vi "HFRR ADV v020 new software.vi"() -> ()   [LabVIEW 2025] (continued)
            n3927 = Concatenate Strings("\",\"ModelNumber\":\"" ("string"), w4967) -> (w4968:string)
            n3928 = Concatenate Strings("\",\"MachineRuntimeHours\":\"" ("string"), w4953) -> (w5071:string)
            n3929 = Concatenate Strings("\",\"MachineRuntimeCycles\":\"", w4962) -> (w5064:string)
            n3930 = Concatenate Strings(w5020, w5016) -> (w5050:string)
            n3931 = Concatenate Strings(w5019, w5006) -> (w5051:string)
            n3932 = Concatenate Strings(w5018, w4988) -> (w5049:string)
            n3933 = Concatenate Strings(w5070, w4968, w5071, w5064) -> (w5073:string)
            n3934 = Concatenate Strings(w5020, w5015) -> (w5047:string)
            n3935 = Concatenate Strings(w5019, w5005) -> (w5046:string)
            n3936 = Concatenate Strings(w5018, w4987) -> (w5048:string)
            n3937 = Concatenate Strings(w5020, w5014) -> (w5042:string)
            n3938 = Concatenate Strings(w5019, w5004) -> (w5043:string)
            n3939 = Concatenate Strings(w5018, w4986) -> (w5041:string)
            n3940 = Concatenate Strings(w5020, w5013) -> (w5039:string)
            n3941 = Concatenate Strings(w5019, w5003) -> (w5038:string)
            n3942 = Concatenate Strings(w5018, w4985) -> (w5040:string)
            n3943 = Concatenate Strings(w5050, w5051, w5049) -> (w5052:string)
            n3944 = Concatenate Strings(w5020, w5012) -> (w5029:string)
            n3945 = Concatenate Strings(w5019, w5002) -> (w5030:string)
            n3946 = Concatenate Strings(w5020, w5011) -> (w5026:string)
            n3947 = Concatenate Strings(w5019, w5001) -> (w5025:string)
            n3948 = Concatenate Strings(w5018, w4984) -> (w5028:string)
            n3949 = Concatenate Strings(w5018, w4983) -> (w5027:string)
            n3950 = Concatenate Strings("{\"SecretKey\":\"", w5067, w5073, "\",\"UUID\" : \"", w5062, "\",\"SensorInformation\":", "[{" ("string")) -> (w5000:string)
            n3951 = Concatenate Strings(w5047, w5046, w5048) -> (w5045:string)
            n3952 = Concatenate Strings(w5042, w5043, w5041) -> (w5044:string)
            n3953 = Concatenate Strings(w5039, w5038, w5040) -> (w5037:string)
            n3954 = Concatenate Strings(w5029, w5030, w5028) -> (w5031:string)
            n3955 = Concatenate Strings(w5026, w5025, w5027) -> (w5024:string)
            n3956 = Concatenate Strings(w5023, w5035, w5052, w4993) -> (w4999:string)
            n3957 = Concatenate Strings(w5023, w5034, w5045, w4993) -> (w4998:string)
            n3958 = Concatenate Strings(w5023, w5033, w5044, w4993) -> (w4997:string)
            n3959 = Concatenate Strings(w5023, w5032, w5037, w4993) -> (w4996:string)
            n3960 = Concatenate Strings(w5023, w5022, w5031, w4993) -> (w4995:string)
            n3961 = Concatenate Strings(w5023, w5021, w5024, "\"}" ("string")) -> (w4994:string)
            n3962 = Concatenate Strings(w5000, w4999, w4998, w4997, w4996, w4995, w4994, "]}" ("string")) -> (w4991:string)
            n3963 = local read "SEN.RUN HRS"() -> (w4958:dbl)
            n3964 = disable-structure shown="Disabled" {
              frame Disabled {
                n3965 = local read "state"() -> (w5077:string[])
                n3966 = Delete From Array(array=w5077, index=0) -> (array with subset deleted=w5075:string[])  [unwired: 1 in, 1 out]
                n3967 = for {
                  N: 6 -> [_]
                  tunnel: w5075 -> [w5088] mode=indexing
                  tunnel: [w5087] -> w5074 mode=indexing
                  n3968 = Equal?(x=w5088, y="Warning") -> (x = y?=w5084:bool)
                  n3969 = Equal?(x=w5088, y="Healthy") -> (x = y?=w5081:bool)
                  n3970 = Select(t="2" ("y"), s=w5084, f="3" ("y")) -> (s? t:f=w5079:string)
                  n3971 = Select(t="1" ("y"), s=w5081, f=w5079) -> (s? t:f=w5087:string)
                }
                "state1" <- w5074
              }
              frame Enabled {
              }
            }
            n3972 = stacked-sequence {
              tunnel: w4991 -> [w5099 _ _]
              tunnel: [_ _ w5115] -> _
              frame #0 {
                (unwired) FALSE ("convert eol (F)")
                w5101 = enum16{"start", "end", "current"}."start" ("pos mode (0:2)")
                n3973 = local read "Path"() -> (w5095:path)
                n3974 = Path To String(path=w5095) -> (string=w5107:string)
                n3975 = Concatenate Strings(w5107, "\\", "Sensor File Name") -> (w5108:string)
                n3976 = local write "standard output 2"(" ") -> ()
                n3977 = String To Path(string=w5108) -> (path=w5098:path)
                n3978 = call <vilib>:"Open_Create_Replace File.vi"("advisory dialog? (display:T)"=FALSE, "function (open:0)"=T32."create or replace", "file path"=w5098) -> ("error out"=w5111:errorcluster, "refnum"=w5110:refnum<file>)  [unwired: 5 in, 2 out]
                n3979 = Set File Position(refnum=w5110, from (0:start)=w5101, error in=w5111) -> (refnum out=w5091:refnum<file>, error out=w5090:errorcluster)  [unwired: 1 in]
                n3980 = Write to Binary File(file (use dialog)=w5091, data=" ", error in=w5090, 5:FALSE ("prepend array or string size? (T)")) -> (refnum out=w5102:refnum<file>, error out=w5103:errorcluster)  [unwired: 2 in, 1 out]
                n3981 = Set File Position(offset (in bytes) (0)=w5101, refnum=w5102, error in=w5103) -> (refnum out=w5094:refnum<file>, error out=w5093:errorcluster)  [unwired: 1 in]
                n3982 = Write to Binary File(file (use dialog)=w5094, data=w5099, error in=w5093, 5:FALSE ("prepend array or string size? (T)")) -> (error out=w5097:errorcluster)  [unwired: 2 in, 2 out]
                n3983 = flat-sequence {
                  tunnel: w5098 -> [w5113]
                  tunnel: w5097 -> [_]
                  frame #0 {
                    n3984 = call <vilib>:"Read Characters From File.vi"("file path (dialog if empty)"=w5113) -> ("character string"=→"Sensor Health JSON string":string)  [unwired: 5 in, 3 out]
                  }
                }
                "SinglePoint  2" <- w5099
              }
              frame #1 {
              }
              frame #2 {
                (unwired) "\"Stored\": true" ("string")
                n3985 = call <vilib>:"System Exec.vi"("run minimized? (F)"=TRUE, "wait until completion? (T)"=TRUE, "working directory"=path "C:/LAB-IQ-NXT", "command line"="C:\\LAB-IQ-NXT\\JPostH.bat") -> ("standard error"=→"Respose From Server 2":string, "standard output"=w5118:string)  [unwired: 4 in, 2 out]
                "standard output 2" <- w5118
                n3986 = Match Pattern(string=w5118, regular expression="JSONH Check String") -> (match substring=w5116:string, offset past match=w5115:i32)  [unwired: 1 in, 2 out]
                n3987 = Equal?(x=w5116, y="JSONH Check String") -> (x = y?=→"Upload \nConfirmed 2":bool)
              }
            }
            n3988 = Divide(x=w4958, y=3600.0 ("f")) -> (x/y=w4951:dbl)
            n3989 = local read "run time"() -> (w5008:string[])
            n3990 = Round To Nearest(number=w4951) -> (nearest integer value=w4950:dbl)
            n3991 = Number To Decimal String(number=w4950) -> (decimal integer string=w4949:string)  [unwired: 1 in]
            n3992 = Index Array(array="Sensor Information", index (col) #1=0 ("disabled index (col)"), index (col) #2=1 ("index (col)"), index (col) #3=2 ("index (col)"), index (col) #4=3 ("index (col)")) -> (element #1=→"Sensor name":string[], element #2=→"model num":string[], element #3=→"run time":string[], element #4=→"state":string[])  [unwired: 4 in]
            n3993 = Insert Into Array(array=w5008, index=1, new element #1=w4949, new element #2=w4949, new element #3=w4949, new element #4=w4949, new element #5=w4949, new element #6=w4949) -> (w4973:string[])
            "run" <- w4973
            n3994 = local read "out"() -> (w4955:string[])
            n3995 = local read "Sensor Information"() -> (w4975:string[][])
            n3996 = Replace Array Subset(array=w4975, new element #1=w4973, index (col) #1=2 ("disabled index (col)"), new element #2=w4955, index (col) #2=3 ("index (col)")) -> (w4974:string[][])  [unwired: 2 in]
            n3997 = local write "Sensor Information"(w4974) -> ()
          }
        }
        n3998 = case shown="True" w4922 {
          frame False {
          }
          frame True {
            n3999 = Equal?(x="FLAG", y=0.0) -> (x = y?=w4939:bool)
            n4000 = case shown="False" w4939 {
              frame False {
                n4001 = Get Date/Time In Seconds() -> (seconds since 1Jan1904=w4945:timestamp)
                n4002 = local read "START 2"() -> (w4943:dbl)
                n4003 = To Double Precision Float(number=w4945) -> (double precision float=w4944:dbl)
                n4004 = Subtract(x=w4944, y=w4943) -> (x-y=→"SENSOR TIME  2":dbl)
              }
              frame True {
                n4005 = Get Date/Time In Seconds() -> (seconds since 1Jan1904=w4947:timestamp)
                n4006 = To Double Precision Float(number=w4947) -> (double precision float=→"START 2":dbl)
                n4007 = local write "FLAG"(100.0 ("FLAG")) -> ()
              }
            }
          }
        }
        n4008 = disable-structure shown="Disabled" {
          disable-tunnel: w4925 -> [w4934 _]
          disable-tunnel: [w4933 _] -> w4924
          frame Disabled {
            n4009 = local read "Json St Flg"() -> (w4932:bool)
            n4010 = case shown="True" w4932 {
              tunnel: w4934 -> [w4935 w4937]
              tunnel: [w4935 w4936] -> w4933
              frame False {
              }
              frame True {
                n4011 = Increment(x=w4937) -> (x+1=w4936:dbl)
                "T cycle" <- w4936
                n4012 = local write "Json St Flg"(FALSE ("Json St Flg")) -> ()
              }
            }
          }
          frame Enabled {
          }
        }
        n4013 = local read "Quit"() -> (w4919:bool)
      }
    }
    frame Enabled {
    }
  }
  n4014 = stacked-sequence {
    tunnel: [w5317] -> w44
    frame #0 {
      w5317 = FALSE ("Upload \nConfirmed")
      n4015 = local write "Upload \nConfirmed"(w5317) -> ()
      n4016 = local write "St Str"("") -> ()
    }
  }
  n4017 = disable-structure shown="Disabled" {
    disable-tunnel: w44 -> [w5318 _]
    frame Disabled {
      n4018 = case shown="True" {
        selector: _ -> [_ _]
        tunnel: w5318 -> [_ w5319]
        frame False {
        }
        frame True {
          n4019 = while {
            tunnel: [w5325] -> _
            tunnel: w5319 -> [_]
            i -> [w5325]
            stop <- w5320 stop-if-true
            n4020 = local read "Json End Flg"() -> (w5324:bool)
            n4021 = Wait (ms)(milliseconds to wait=u32 20 ("Refresh Rate (ms)")) -> ()  [unwired: 1 out]
            n4022 = local read "refresh flag"() -> (w5321:bool)
            n4023 = local read "RUN"() -> (w5322:bool)
            n4024 = And(x=w5322, y=w5321) -> (x .and. y?=w5323:bool)
            n4025 = Or(x=w5323, y=w5324) -> (x .or. y?=w5326:bool)
            "AR Led" <- w5326
            n4026 = case shown="True" w5326 {
              frame False {
              }
              frame True {
                w5343 = "\",\""
                n4027 = local read "UUID"() -> (w5341:string)
                n4028 = local write "refresh flag"(FALSE ("refresh flag")) -> ()
                n4029 = local read "time"() -> (w5330:dbl)
                n4030 = Multiply(x=w5330, y=60.0) -> (x*y=w5329:dbl)
                n4031 = Concatenate Strings("UUID\" : \"", w5341, "\"}") -> (w5344:string)
                n4032 = Number To Fractional String(number=w5329, width (-)=i16 10, precision (6)=i16 4) -> (F-format string=w5358:string)  [unwired: 1 in]
                n4033 = Concatenate Strings("{", "\"Time\":\"", w5358, w5343) -> (w5353:string)
                n4034 = stacked-sequence {
                  tunnel: w5343 -> [w5406 w5414 w5421 w5429 w5437 w5446 w5453]
                  tunnel: [w5407 _ _ _ _ _ _] -> w5357
                  tunnel: [_ w5415 _ _ _ _ _] -> w5356
                  tunnel: [_ _ w5422 _ _ _ _] -> w5355
                  tunnel: [_ _ _ w5431 _ _ _] -> w5354
                  tunnel: w5344 -> [_ _ _ _ _ _ w5464]
                  tunnel: [_ _ _ _ _ _ w5463] -> w5340
                  tunnel: [_ _ _ _ _ w5443 _] -> w5339
                  tunnel: [_ _ _ _ w5436 _ _] -> w5338
                  frame #0 {
                    n4035 = local read "NORMAL LOAD"() -> (w5405:dbl)
                    n4036 = Number To Fractional String(number=w5405, width (-)=i16 10, precision (6)=i16 4) -> (F-format string=w5408:string)  [unwired: 1 in]
                    n4037 = Concatenate Strings("NormalLoad\":\"", w5408, w5406) -> (w5407:string)
                  }
                  frame #1 {
                    n4038 = local read "Temp"() -> (w5413:dbl)
                    n4039 = Number To Fractional String(number=w5413, width (-)=i16 10, precision (6)=i16 4) -> (F-format string=w5416:string)  [unwired: 1 in]
                    n4040 = Concatenate Strings("Temperature\":\"", w5416, w5414) -> (w5415:string)
                  }
                  frame #2 {
                    n4041 = local read "cof"() -> (w5419:dbl)
                    n4042 = Number To Fractional String(number=w5419, width (-)=i16 10, precision (6)=i16 4) -> (F-format string=w5423:string)  [unwired: 1 in]
                    n4043 = Concatenate Strings("FrictionalForce\":\"", w5423, w5421) -> (w5422:string)
                  }
                  frame #3 {
                    n4044 = local read "Set Hz"() -> (w5427:dbl)
                    n4045 = Multiply(x=w5427, y=60.0) -> (x*y=w5426:dbl)
                    n4046 = Number To Fractional String(number=w5426, width (-)=i16 10, precision (6)=i16 4) -> (F-format string=w5432:string)  [unwired: 1 in]
                    n4047 = Concatenate Strings("Speed\":\"", w5432, w5429) -> (w5431:string)
                  }
                  frame #4 {
                    n4048 = local read item#-1() -> (w5435)
                    n4049 = Number To Fractional String(number=w5435, width (-)=i16 10, precision (6)=i16 4) -> (F-format string=w5439:string)  [unwired: 1 in]
                    n4050 = Concatenate Strings("LinearDeformation\":\"", w5439, w5437) -> (w5436:string)
                  }
                  frame #5 {
                    n4051 = local read "AIR TEMP"() -> (w5442:dbl)
                    n4052 = local read "Json St Flg"() -> (w5444:bool)
                    n4053 = local read "Json End Flg"() -> (w5445:bool)
                    n4054 = Number To Fractional String(number=w5442, width (-)=i16 10, precision (6)=i16 4) -> (F-format string=w5448:string)  [unwired: 1 in]
                    n4055 = Concatenate Strings("Vibration\":\"", w5448, w5446) -> (w5443:string)
                    n4056 = And(x=w5444, y=w5445) -> ()  [unwired: 1 out]
                  }
                  frame #6 {
                    n4057 = local read "Json End Flg"() -> (w5452:bool)
                    n4058 = Get Date/Time In Seconds() -> (seconds since 1Jan1904=w5460:timestamp)
                    n4059 = local read "Json St Flg"() -> (w5451:bool)
                    n4060 = To Double Precision Float(number=w5460) -> (double precision float=w5459:dbl)
                    n4061 = Subtract(x=w5459, y=2082844800.0) -> (x-y=w5457:dbl)
                    n4062 = Number To Fractional String(number=w5457, width (-)=i16 12, precision (6)=i16 0) -> (F-format string=w5454:string)  [unwired: 1 in]
                    n4063 = case shown="True" w5452 {
                      tunnel: ["" w5467] -> w5461
                      tunnel: w5454 -> [_ w5468]
                      tunnel: w5453 -> [_ w5466]
                      frame False {
                      }
                      frame True {
                        n4064 = local write "Json End Flg"(FALSE ("Json St Flg")) -> ()
                        n4065 = Concatenate Strings("End\": \"", w5468, w5466) -> (w5467:string)
                      }
                    }
                    n4066 = case shown="True" w5451 {
                      tunnel: [w5471 w5474] -> w5462
                      tunnel: w5454 -> [_ w5475]
                      tunnel: w5453 -> [_ w5472]
                      frame False {
                        n4067 = local read "St Str"() -> (w5471:string)
                      }
                      frame True {
                        n4068 = Concatenate Strings("Start\":\"", w5475, w5472) -> (w5474:string)
                        "St Str" <- w5474
                        n4069 = local write "Json St Flg"(FALSE ("Json St Flg")) -> ()
                      }
                    }
                    n4070 = Concatenate Strings(w5462, w5461, w5464) -> (w5463:string)
                  }
                }
                n4071 = local read "FILE"() -> (w5332:string)
                n4072 = Concatenate Strings("\",\"OperatorID\":\"" ("string"), "Operator ID") -> (w5335:string)
                n4073 = Concatenate Strings("\",\"DatasetTitle\":\"" ("string"), w5332) -> (w5334:string)
                n4074 = Concatenate Strings("\",\"SerialNumber\":\"" ("string"), "Serial No") -> (w5364:string)
                n4075 = Concatenate Strings("\",\"ModelNumber\":\"" ("string"), "Model No") -> (w5363:string)
                n4076 = Concatenate Strings(w5364, w5363) -> (w5346:string)
                n4077 = Concatenate Strings("{\"SecretKey\":\"", "Secret Key", w5346, w5335, w5334, "\",\"Samples\":[") -> (w5351:string)
                n4078 = Concatenate Strings(w5353, w5357, w5356, w5355, w5354, w5338, w5339, w5340) -> (w5352:string)
                n4079 = Concatenate Strings(w5351, w5352, "]}") -> (w5350:string)
                n4080 = stacked-sequence {
                  tunnel: w5350 -> [w5379 _ _]
                  tunnel: [_ _ w5396] -> _
                  frame #0 {
                    (unwired) FALSE ("convert eol (F)")
                    w5381 = enum16{"start", "end", "current"}."start" ("pos mode (0:2)")
                    n4081 = Path To String(path="Path") -> (string=w5387:string)
                    n4082 = Concatenate Strings(w5387, "\\", "Data File Name") -> (w5389:string)
                    n4083 = local write "standard output"(" ") -> ()
                    n4084 = String To Path(string=w5389) -> (path=w5378:path)
                    n4085 = call <vilib>:"Open_Create_Replace File.vi"("advisory dialog? (display:T)"=FALSE, "function (open:0)"=T32."create or replace", "file path"=w5378) -> ("error out"=w5392:errorcluster, "refnum"=w5391:refnum<file>)  [unwired: 5 in, 2 out]
                    n4086 = Set File Position(refnum=w5391, from (0:start)=w5381, error in=w5392) -> (refnum out=w5372:refnum<file>, error out=w5371:errorcluster)  [unwired: 1 in]
                    n4087 = Write to Binary File(file (use dialog)=w5372, data=" ", error in=w5371, 5:FALSE ("prepend array or string size? (T)")) -> (refnum out=w5382:refnum<file>, error out=w5383:errorcluster)  [unwired: 2 in, 1 out]
                    n4088 = Set File Position(offset (in bytes) (0)=w5381, refnum=w5382, error in=w5383) -> (refnum out=w5375:refnum<file>, error out=w5374:errorcluster)  [unwired: 1 in]
                    n4089 = Write to Binary File(file (use dialog)=w5375, data=w5379, error in=w5374, 5:FALSE ("prepend array or string size? (T)")) -> (error out=w5377:errorcluster)  [unwired: 2 in, 2 out]
                    n4090 = flat-sequence {
                      tunnel: w5378 -> [w5394]
                      tunnel: w5377 -> [_]
                      frame #0 {
                        n4091 = call <vilib>:"Read Characters From File.vi"("file path (dialog if empty)"=w5394) -> ("character string"=→"JSON string":string)  [unwired: 5 in, 3 out]
                      }
                    }
                    "SinglePoint" <- w5379
                  }
                  frame #1 {
                  }
                  frame #2 {
                    (unwired) "\"Stored\": true" ("string")
                    n4092 = call <vilib>:"System Exec.vi"("run minimized? (F)"=TRUE, "wait until completion? (T)"=TRUE, "working directory"=path "C:/LAB-IQ-NXT", "command line"="C:\\LAB-IQ-NXT\\JPost.bat") -> ("standard error"=→"Respose From Server":string, "standard output"=w5399:string)  [unwired: 4 in, 2 out]
                    "standard output" <- w5399
                    n4093 = Match Pattern(string=w5399, regular expression="JSON Check String") -> (match substring=w5397:string, offset past match=w5396:i32)  [unwired: 1 in, 2 out]
                    n4094 = Equal?(x=w5397, y="JSON Check String") -> (x = y?=→"Upload \nConfirmed":bool)
                  }
                }
              }
            }
            n4095 = local read "Quit"() -> (w5320:bool)
          }
        }
      }
    }
    frame Enabled {
    }
  }
  n4096 = disable-structure shown="Disabled" {
    disable-tunnel: _ -> [w5482 _]
    frame Disabled {
      n4097 = while {
        shift-right: [w5490] -> w5478
        shift-left: _ -> [w5491]
        shift-right: [w5488] -> w5479
        shift-left: errorcluster {"status"=TRUE, "code"=0, "source"="Init"} ("error out") -> [w5489]
        shift-right: [w5486] -> _
        shift-left: "" -> [w5487]
        tunnel: [w5484] -> _
        tunnel: w5482 -> [_]
        i -> [w5484]
        stop <- w5483 stop-if-true
        n4098 = flat-sequence {
          tunnel: [w5492] -> w5485
          frame #0 {
            n4099 = Wait (ms)(milliseconds to wait=10.0 ("Delay")) -> (millisecond timer value=w5492:u32)
          }
        }
        n4100 = case shown="No Error" w5489 {
          selector: w5489 -> [w5522 w5641]
          tunnel: [w5505 w5643] -> w5490
          tunnel: [w5504 w5642] -> w5488
          tunnel: w5491 -> [w5523 w5635]
          tunnel: w5487 -> [w5503 w5634]
          tunnel: [w5502 w5634] -> w5486
          tunnel: w5485 -> [_ _]
          frame No Error {
            n4101 = Concatenate Strings("\r", "\n") -> (w5514:string)  [unwired: 1 in]
            n4102 = case shown="True" w5515 {
              tunnel: w5523 -> [w5547 w5554]
              tunnel: w5522 -> [w5546 w5553]
              tunnel: [w5547 w5552] -> w5521
              tunnel: [w5546 w5551] -> w5501
              tunnel: w5514 -> [_ w5550]
              frame False {
              }
              frame True {
                n4103 = VISA Write(VISA resource name=w5554, write buffer=w5550, error in (no error)=w5553) -> (VISA resource name out=w5552:refnum<visa-resource-name>, error out=w5551:errorcluster)  [unwired: 1 out]
                n4104 = local write "Read String"("") -> ()
                n4105 = local write item#-1(FALSE) -> ()
              }
            }
            n4106 = property class="Instr"(reference=w5521, error in=w5501) -> (reference out=w5520:refnum<visa-resource-name>, error out=w5519:errorcluster, "Serial Settings:Number of Bytes at Serial Port"=w5518:u32)
            n4107 = Greater?(x=w5518, y=u32 100) -> (0:w5516:bool)
            n4108 = case shown="True" w5516 {
              tunnel: w5520 -> [w5557 w5581]
              tunnel: w5519 -> [w5556 w5580]
              tunnel: w5518 -> [_ w5579]
              tunnel: [w5557 w5578] -> w5507
              tunnel: [w5556 w5577] -> w5506
              tunnel: w5503 -> [w5555 w5576]
              tunnel: [w5555 ""] -> w5502
              frame False {
              }
              frame True {
                w5566 = u32 6 ("y")
                # "Page 84 of \nmanual"
                n4109 = VISA Read(VISA resource name=w5581, byte count=w5579, error in (no error)=w5580) -> (VISA resource name out=w5578:refnum<visa-resource-name>, read buffer=w5574:string, error out=w5577:errorcluster)  [unwired: 1 out]
                n4110 = while {
                  tunnel: w5574 -> [w5630]
                  tunnel: [w5626] -> w5568 mode=indexing
                  tunnel: [w5620] -> w5572 mode=indexing
                  tunnel: [w5618] -> _
                  i -> [w5618]
                  stop <- w5623 stop-if-true
                  n4111 = String Subset(string=w5630, offset (0)=w5618) -> (substring=w5625:string)  [unwired: 1 in]
                  n4112 = String To Byte Array(string=w5625) -> (unsigned byte array=w5629:u8[])
                  n4113 = String Length(string=w5625) -> (length=w5624:i32)
                  n4114 = Index Array(array=w5629) -> (element=w5628:u8)  [unwired: 1 in]
                  n4115 = Equal To 0?(x=w5624) -> (x = 0?=w5623:bool)
                  n4116 = Number To Boolean Array(number=w5628) -> (Boolean array=w5622:bool[])
                  n4117 = Reverse 1D Array(array=w5622) -> (reversed array=w5621:bool[])
                  n4118 = And(x=w5622, y=bool[] [FALSE, FALSE, FALSE, FALSE, FALSE, FALSE, TRUE, TRUE] ("Boolean array")) -> (x .and. y?=w5626:bool[])
                  n4119 = And(x=w5621, y=bool[] [FALSE, FALSE, TRUE, TRUE, TRUE, TRUE, TRUE, TRUE] ("Boolean array")) -> (x .and. y?=w5620:bool[])
                }
                n4120 = Concatenate Strings(w5576, w5574) -> (→"Read String":string)
                n4121 = while {
                  tunnel: w5568 -> [w5617] mode=indexing
                  tunnel: [w5613] -> w5571
                  i -> [w5613]
                  stop <- w5614 stop-if-true
                  n4122 = Search 1D Array(1D array=w5617, element=TRUE) -> (index of element=w5615:i32)  [unwired: 1 in]
                  n4123 = Less Than 0?(x=w5615) -> (x < 0?=w5614:bool)
                }
                n4124 = Delete From Array(array=w5572, length=w5571, index (row)=0) -> (array with subset deleted=w5567:bool[][])  [unwired: 1 in, 1 out]
                n4125 = Array Size(array=w5567) -> (size(s)=w5569:i32[])
                n4126 = Index Array(array=w5569) -> (element=w5561:i32)  [unwired: 1 in]
                n4127 = Greater?(x=w5561, y=w5566) -> (0:w5564:bool)
                n4128 = Subtract(x=w5561, y=w5566) -> (x-y=w5565:u32)
                n4129 = Select(t=w5565, s=w5564, f=u32 0) -> (s? t:f=w5562:u32)
                n4130 = while {
                  tunnel: w5567 -> [w5600]
                  tunnel: [w5602] -> w5560 mode=indexing
                  tunnel: w5562 -> [w5584]
                  i -> [w5601]
                  stop <- w5599 stop-if-true
                  w5591 = 6 ("index")
                  w5590 = 2 ("length")
                  # "Page 65 of \nmanual"
                  n4131 = Multiply(x=u32 3 ("y"), y=w5601) -> (x*y=w5598:u32)
                  n4132 = Divide(x=u32 102 ("y"), y=u32 65520) -> (x/y=w5608:dbl)
                  n4133 = Greater Or Equal?(x=w5598, y=w5584) -> (x >= y?=w5599:bool)
                  n4134 = Index Array(array=w5600, index (row) #1=w5598) -> (element #1=w5596:bool[], element #2=w5595:bool[], element #3=w5594:bool[])  [unwired: 5 in]
                  n4135 = Reverse 1D Array(array=w5596) -> (reversed array=w5589:bool[])
                  n4136 = Reverse 1D Array(array=w5595) -> (reversed array=w5593:bool[])
                  n4137 = Reverse 1D Array(array=w5594) -> (reversed array=w5592:bool[])
                  n4138 = Delete From Array(array=w5589, length=w5590, index=w5591) -> (array with subset deleted=w5585:bool[])  [unwired: 1 out]
                  n4139 = Delete From Array(array=w5593, length=w5590, index=w5591) -> (array with subset deleted=w5586:bool[])  [unwired: 1 out]
                  n4140 = Delete From Array(array=w5592, length=w5590, index=w5591) -> (array with subset deleted=w5587:bool[])  [unwired: 1 out]
                  n4141 = Insert Into Array(array=bool[] [] ("Boolean array"), new element #1=w5585, new element #2=w5586, new element #3=w5587) -> (w5588:bool[])  [unwired: 1 in]
                  n4142 = Boolean Array To Number(Boolean array=w5588) -> (number=w5597:u32)
                  n4143 = Multiply(x=w5608, y=w5597) -> (x*y=w5607:dbl)
                  n4144 = Decrement(x=w5607) -> (x-1=w5606:dbl)
                  n4145 = Divide(x=w5606, y=u32 100) -> (x/y=w5604:dbl)
                  n4146 = Multiply(x=w5604, y=u32 10) -> (x*y=w5602:dbl)
                }
                n4147 = Delete From Array(array=w5560) -> (array with subset deleted=w5559:dbl[])  [unwired: 2 in, 1 out]
                "Waveform Graph 5" <- w5559
                "Waveform Chart 3" <- w5559
                n4148 = call-poly <vilib>:"Mean.vi"("X"=w5559) -> ("mean"=w5558:dbl)  [unwired: 1 out]
                n4149 = case shown="True" {
                  selector: _ -> [_ _]
                  tunnel: w5558 -> [_ w5583]
                  frame False {
                  }
                  frame True {
                    n4150 = local write item#-1(FALSE ("Zero 4")) -> ()
                    "z_measure" <- w5583
                  }
                }
              }
            }
            n4151 = local read item#-1() -> (w5498)
            n4152 = local read item#-1() -> (w5497)
            n4153 = local read item#-1() -> (w5499)
            n4154 = local read item#-1() -> (w5496)
            n4155 = case shown="True" w5494 {
              tunnel: w5498 -> [_ w5526]
              tunnel: w5499 -> [_ w5525]
              frame False {
              }
              frame True {
                n4156 = Build Array(w5526, w5525) -> (w5524:void[])
                n4157 = local read item#-1() -> (w5529)
                n4158 = Build Array (concatenate)(w5529, w5524) -> (w5527:void[])
                n4159 = local write item#-1(w5527) -> ()
                n4160 = local write item#-1(FALSE ("Boolean 8")) -> ()
              }
            }
            n4161 = call "Build XY Graph"("Enable"=w5496, "Reset"=w5497, "Y Input"=w5499, "X Input"=w5498) -> ("XY Graph"=w5495:cluster{"Y":dbl[], "Y":dbl[]}[])  [unwired: 6 in, 1 out]
            n4162 = case shown="True" {
              selector: _ -> [_ _]
              frame False {
              }
              frame True {
                n4163 = local read item#-1() -> (w5530)
                n4164 = Index Array(array=w5530, index (col) #1=0 ("disabled index (col)"), index (col) #2=1 ("index (col)")) -> (element #1=w5532, element #2=w5531)  [unwired: 2 in]
                n4165 = call <vilib>:"Linear Fit.vi"("Y"=w5532, "X"=w5531) -> ()  [unwired: 9 in, 5 out]
                n4166 = local write item#-1(FALSE ("Boolean 9")) -> ()
              }
            }
            n4167 = case shown="True" {
              selector: _ -> [_ _]
              frame False {
              }
              frame True {
                n4168 = local write item#-1(dbl[][] [] ("Captured Values")) -> ()
                n4169 = local write item#-1(FALSE ("Boolean 7")) -> ()
              }
            }
            n4170 = Concatenate Strings("\r", "\n") -> (w5509:string, w5508:string)
            n4171 = case shown="True" w5500 {
              tunnel: w5507 -> [w5539 w5545]
              tunnel: w5506 -> [w5538 w5544]
              tunnel: [w5539 w5543] -> w5505
              tunnel: [w5538 w5542] -> w5504
              tunnel: w5509 -> [_ w5541]
              frame False {
              }
              frame True {
                n4172 = VISA Write(VISA resource name=w5545, write buffer=w5541, error in (no error)=w5544) -> (VISA resource name out=w5543:refnum<visa-resource-name>, error out=w5542:errorcluster)  [unwired: 1 out]
                n4173 = local write item#-1(FALSE ("WRITE")) -> ()
              }
            }
          }
          frame Error {
            w5633 = u16 10 items=["1.0"=10, "1.5"=15, "2.0"=20] ("stop bits (10: 1 bit)")
            n4174 = Wait (ms)(milliseconds to wait=u32 20) -> ()  [unwired: 1 out]
            n4175 = VISA Close(VISA resource name=w5635, error in (no error)=w5641) -> (error out=w5640:errorcluster)
            n4176 = call <vilib>:"Clear Errors.vi"("error in (no error)"=w5640) -> ("error out"=w5639:errorcluster)  [unwired: 5 in, 1 out]
            n4177 = call-poly "VISA Configure Serial Port"("timeout (10sec)"=u32 200, "Enable Termination\nChar (T)"=TRUE ("Enable Termination\nChar (T)"), "baud rate (9600)"=u32 921600, "error in (no error)"=w5639, "stop bits (10: 1 bit)"=w5633) -> ("VISA resource name"=w5631:refnum<visa-resource-name>, "VISA resource name out"=w5643:refnum<visa-resource-name>, "error out"=w5642:errorcluster)  [unwired: 8 in]
          }
        }
        n4178 = local read "Quit"() -> (w5483:bool)
      }
      n4179 = VISA Close(VISA resource name=w5478, error in (no error)=w5479) -> (error out=w5477:errorcluster)
      n4180 = call <vilib>:"Clear Errors.vi"("error in (no error)"=w5477) -> ()  [unwired: 5 in, 2 out]
    }
    frame Enabled {
    }
  }
  n4181 = disable-structure shown="Disabled" {
    disable-tunnel: _ -> [w5648 _]
    frame Disabled {
      n4182 = while {
        tunnel: [w5655] -> _
        shift-right: [w5652] -> w5645
        shift-left: _ -> [w5654]
        shift-right: [w5653] -> w5646
        shift-left: errorcluster {"status"=TRUE, "code"=0, "source"="Init"} ("error out") -> [w5651]
        tunnel: w5648 -> [_]
        i -> [w5655]
        stop <- w5649 stop-if-true
        n4183 = flat-sequence {
          tunnel: w5651 -> [w5746]
          tunnel: [w5746] -> w5650
          frame #0 {
            n4184 = Wait (ms)(milliseconds to wait=u32 50) -> ()  [unwired: 1 out]
          }
        }
        n4185 = case shown="No Error" w5650 {
          selector: w5650 -> [w5696 w5739]
          tunnel: w5654 -> [w5695 w5738]
          tunnel: [w5662 w5729] -> w5653
          tunnel: [w5663 w5737] -> w5652
          frame No Error {
            w5689 = T33 {"Mode"=enum."RTU", "Slave Address"=1} ("Serial Parameters")
            n4186 = call-poly <vilib>:"MB Serial Master Query (poly).vi"("VISA resource name"=w5695, "Starting Address"=i16 1000, "Quantity"=u16 1, "Timeout"=u32 1000, "error in"=w5696, "Serial Parameters"=w5689) -> ("VISA resource name out"=w5690:refnum<visa-resource-name>, "Input Registers"=w5692:u16[], "error out"=w5688:errorcluster)  [unwired: 10 in, 1 out]
            n4187 = Random Number (0-1)() -> (number: 0 to 1=w5677:dbl)
            n4188 = Index Array(array=w5692, index=0) -> (element=w5687:u16)
            n4189 = Subtract(x=w5677, y=0.5) -> (x-y=w5676:dbl)
            n4190 = Divide(x=w5687, y=10 ("index")) -> (x/y=w5681:dbl)
            n4191 = Multiply(x=w5676, y=0.5) -> (x*y=w5675:dbl)
            n4192 = Add(x=w5681, y=w5675) -> (x+y=w5680:dbl)
            n4193 = local read "Amb temp"() -> (w5664:dbl)
            n4194 = Multiply(x=w5680, y=0.2) -> (x*y=w5684:dbl)
            n4195 = Multiply(x=w5664, y=0.8) -> (x*y=w5682:dbl)
            n4196 = Add(x=w5684, y=w5682) -> (x+y=w5665:dbl)
            n4197 = local read "set temp old"() -> (w5659:dbl)
            n4198 = local write "Amb temp"(w5665) -> ()
            n4199 = Select(t="SetTemp 2", s="Heater", f=100.0) -> (s? t:f=w5660:dbl)
            n4200 = Not Equal?(x=w5660, y=w5659) -> (x != y?=w5658:bool)
            n4201 = case shown="True" w5658 {
              tunnel: w5690 -> [w5724 w5726]
              tunnel: [w5723 w5726] -> w5670
              tunnel: w5688 -> [w5722 w5725]
              tunnel: [w5721 w5725] -> w5668
              tunnel: w5660 -> [w5716 _]
              tunnel: w5689 -> [w5718 w5727]
              tunnel: [w5718 w5727] -> w5671
              frame True {
                n4202 = Multiply(x=w5716, y=10 ("index")) -> (x*y=w5715:dbl)
                n4203 = call-poly <vilib>:"MB Serial Master Query (poly).vi"("VISA resource name"=w5724, "Address"=u16 0, "Holding Register"=w5715, "Timeout"=u32 1000, "error in"=w5722, "Serial Parameters"=w5718) -> ("VISA resource name out"=w5723:refnum<visa-resource-name>, "error out"=w5721:errorcluster)  [unwired: 11 in, 1 out]
                "set temp old" <- w5716
              }
              frame False {
              }
            }
            n4204 = flat-sequence {
              tunnel: [w5697] -> _
              tunnel: [w5697] -> w5667
              tunnel: w5668 -> [w5697]
              frame #0 {
                n4205 = Wait (ms)(milliseconds to wait=u32 100) -> ()  [unwired: 1 out]
              }
            }
            n4206 = call "Elapsed Time12"("Time Target (s)"=2.0, "Auto Reset"=TRUE) -> ("Time has Elapsed"=w5672:bool)  [unwired: 10 in, 7 out]
            n4207 = case shown="True" w5672 {
              tunnel: w5671 -> [w5701 w5714]
              tunnel: [w5701 w5714] -> _
              tunnel: [w5700 w5712] -> w5663
              tunnel: w5670 -> [w5700 w5713]
              tunnel: [w5699 w5710] -> w5662
              tunnel: w5667 -> [w5699 w5711]
              frame False {
              }
              frame True {
                n4208 = call-poly <vilib>:"MB Serial Master Query (poly).vi"("VISA resource name"=w5713, "Starting Address"=i16 1003 ("Addr"), "Quantity"=u16 1, "Timeout"=u32 1000, "error in"=w5711, "Serial Parameters"=w5714) -> ("VISA resource name out"=w5712:refnum<visa-resource-name>, "Input Registers"=w5707:u16[], "error out"=w5710:errorcluster)  [unwired: 10 in, 1 out]
                n4209 = Index Array(array=w5707, index=0) -> (element=w5706:u16)
                n4210 = Divide(x=w5706, y=u16 10) -> (x/y=w5702:dbl)
                n4211 = local write "set temp old"(w5702) -> ()
                n4212 = local write "SetTemp"(w5702) -> ()
              }
            }
            "Error Code" <- w5662
            n4213 = Unbundle(w5662) -> ("status"=→"TK4 status":bool)  [unwired: 2 out]
            "SetTemp" <- "SetTemp 2"
          }
          frame Error {
            w5741 = u16 0 items=["None", "Odd", "Even", "Mark", "Space"] ("Parity")
            w5742 = u16 0 items=["None", "XON/XOFF", "RTS/CTS", "XON/XOFF & RTS/CTS", "DTR/DSR", "XON/XOFF & DTR/DSR"] ("Flow Control")
            n4214 = VISA Clear(VISA resource name=w5738, error in (no error)=w5739) -> (VISA resource name out=w5732:refnum<visa-resource-name>, error out=w5730:errorcluster)
            n4215 = VISA Close(VISA resource name=w5732, error in (no error)=w5730) -> (error out=w5731:errorcluster)
            n4216 = call <vilib>:"Clear Errors.vi"("error in (no error)"=w5731) -> ("error out"=w5740:errorcluster)  [unwired: 5 in, 1 out]
            n4217 = Unbundle By Name(T33 {"Mode"=enum."RTU", "Slave Address"=1} ("input cluster")) -> ("Mode"=w5743:enum16{"RTU", "ASCII"})
            n4218 = call <vilib>:"MB Serial Init.vi"("Timeout"=u32 100, "Flow Control"=w5742, "Mode"=w5743, "error in (no error)"=w5740, "Parity"=w5741, "Baud Rate"=u32 9600, "VISA resource name"="Lubrication System COM Port :") -> ("error out"=w5729:errorcluster, "VISA resource name out"=w5737:refnum<visa-resource-name>)  [unwired: 3 in]
            n4219 = local write "set temp old"(0.0 ("set temp old")) -> ()
            n4220 = Unbundle(w5729) -> ("status"=w5728:bool)  [unwired: 2 out]
            n4221 = case shown="True" w5728 {
              selector: w5728 -> [_ w5745]
              frame False {
              }
              frame True {
                n4222 = local write "TK4 status"(w5745) -> ()
              }
            }
          }
        }
        n4223 = local read "Quit"() -> (w5649:bool)
      }
      n4224 = VISA Close(VISA resource name=w5645, error in (no error)=w5646) -> (error out=w5644:errorcluster)
      n4225 = call <vilib>:"Clear Errors.vi"("error in (no error)"=w5644) -> ()  [unwired: 5 in, 2 out]
    }
    frame Enabled {
    }
  }
